vi "rest invent.vi"(8 "error in (no error)":errorcluster, 9 "Numeric":u16, 10 "Prods":string[][](array[string]), 11 "Coca Actor in":refnum<class "Coca Actor.lvclass">) -> (0 "error out":errorcluster, 3 "Coca Actor out":refnum<class "Coca Actor.lvclass">)   [LabVIEW 2020, in "Coca Actor.lvlib" / "Coca Actor.lvclass"]
uses:
  Coca Actor.lvclass
  C:/Program Files (x86)/National Instruments/LabVIEW 2020/vi.lib/ActorFramework/Actor/Actor.lvclass
  Coca Actor.lvclass/Coca Actor.ctl
  <vilib>/ActorFramework/Actor/Actor.lvclass/Actor.ctl
  UI Actor Messages/Compras Msg/Compras Msg.lvclass/Compras Msg.ctl
  <vilib>/ActorFramework/Message Enqueuer/Message Enqueuer.lvclass/Message Enqueuer.ctl
  <vilib>/ActorFramework/Message Enqueuer/Enqueue.vi
  UI Actor Messages/Compras Msg/Compras Msg.lvclass
  C:/Program Files (x86)/National Instruments/LabVIEW 2020/vi.lib/ActorFramework/Message/Message.lvclass
  <vilib>/ActorFramework/Message Priority Queue/Priority Enqueue.vi
  <vilib>/ActorFramework/Actor/Actor.lvclass
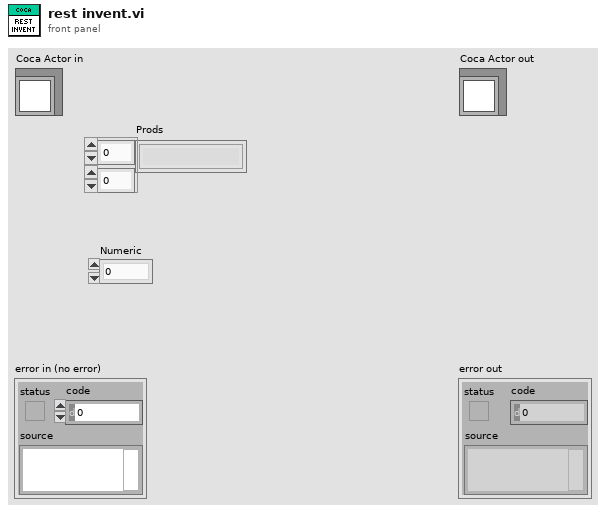
[diagram p1: front panel]
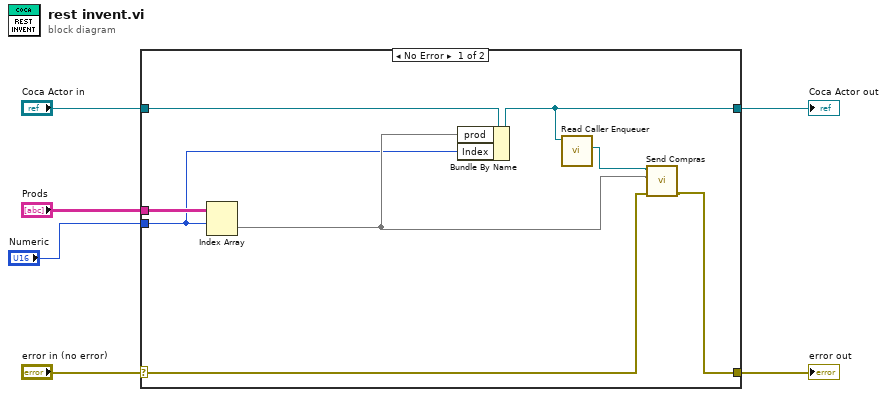
[diagram p0: block diagram]
diagram:
  n1 = case shown="No Error" "error in (no error)" {
    selector: "error in (no error)" -> [w9 w16]
    tunnel: [w8 w16] -> w5
    tunnel: [w12 w15] -> w3
    tunnel: "Coca Actor in" -> [w13 w15]
    tunnel: "Prods" -> [w14 _]
    tunnel: "Numeric" -> [w7 _]
    frame No Error {
      n2 = Index Array "Index Array"(array=w14, index (row)=w7) -> (element=w10:string[])  [unwired: 1 in]
      n3 = Bundle By Name(cluster=w13, "prod"=w10, "Index"=w7) -> (w12:refnum<class "Coca Actor.lvclass">)
      n4 = call <vilib>:"Read Caller Enqueuer.vi"("Actor"=w12) -> ("Caller Enqueuer"=w11:refnum<class "Message Enqueuer.lvclass">)  [unwired: 10 in]
      n5 = call "Send Compras.vi"("error in (no error)"=w9, "product"=w10, "Message Enqueuer"=w11) -> ("error out"=w8:errorcluster)  [unwired: 7 in, 1 out]
    }
    frame Error {
    }
  }
  "error out" <- w5
  "Coca Actor out" <- w3
